vi "PotentiometerVoltage.vi"() -> ()   [LabVIEW 2018]
panel:
  in  "Calibration Voltage":dbl
  out "Mass G":dbl
  out "Waveform Chart":dbl(graph)
  in  "stop":bool
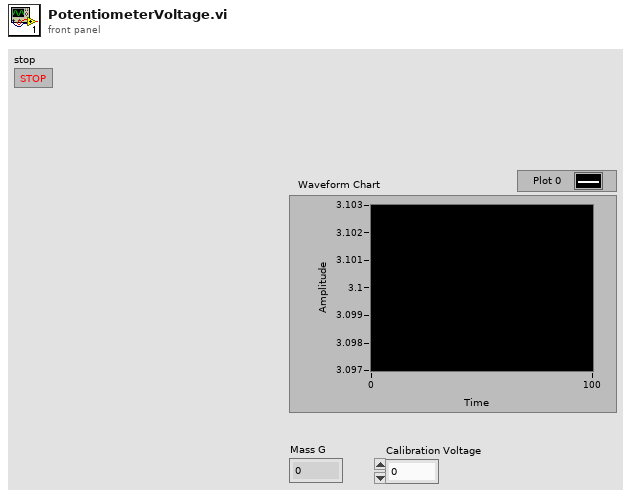
[diagram p1: front panel]
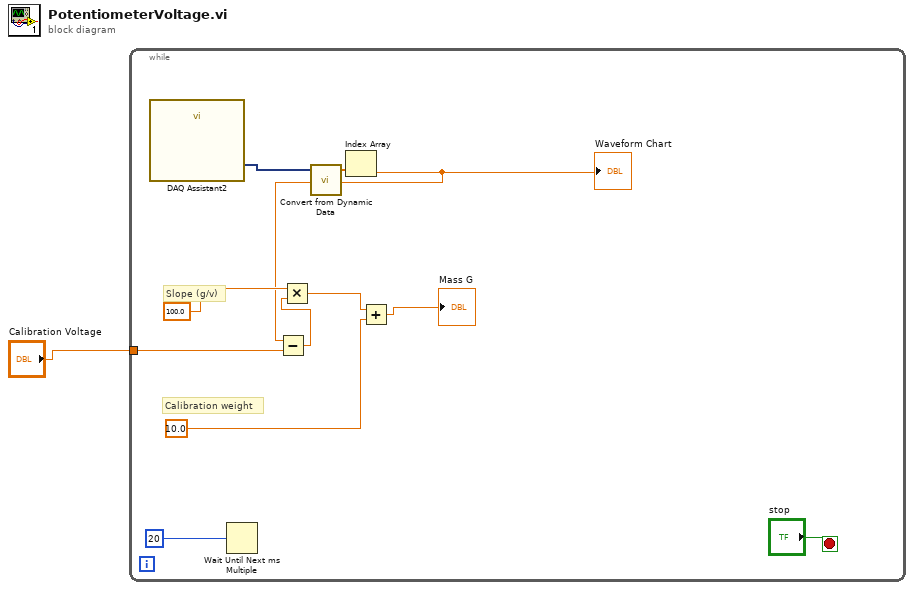
[diagram p0: block diagram]
diagram:
  n1 = while {
    tunnel: "Calibration Voltage" -> [w3]
    stop <- "stop" stop-if-true
    # "Calibration weight"
    # "Slope (g/v)"
    n2 = call "DAQ Assistant2"() -> ("data"=w11:dynamicdata)  [unwired: 17 in, 2 out]
    n3 = Wait Until Next ms Multiple(millisecond multiple=20) -> ()  [unwired: 1 out]
    n4 = call "Convert from Dynamic Data"("Dynamic Data Type"=w11) -> ("Array"=w10:dbl[])  [unwired: 3 in]
    n5 = Index Array(array=w10) -> (element=w2:dbl)  [unwired: 1 in]
    "Waveform Chart" <- w2
    n6 = Subtract(x=w2, y=w3) -> (x-y=w7:dbl)
    n7 = Multiply(x=100.0, y=w7) -> (x*y=w6:dbl)
    n8 = Add(x=w6, y=10.0) -> (x+y=→"Mass G":dbl)
  }
